vi "addmmWaveRefnums.vi"(8 "error in (no error)":errorcluster, 9 "mmWave motion ctrls":T1, 11 "UI ExecutionCtrls in":refnum<class "UI ExecutionCtrls.lvclass">) -> (0 "error out":errorcluster, 3 "UI ExecutionCtrls out":refnum<class "UI ExecutionCtrls.lvclass">)   [LabVIEW 2018, in "UI ExecutionCtrls.lvclass"]
uses:
  UI ExecutionCtrls.lvclass
  mmWaveMotionCrtlRefs.ctl
  UI ExecutionCtrls.lvclass/UI ExecutionCtrls.ctl
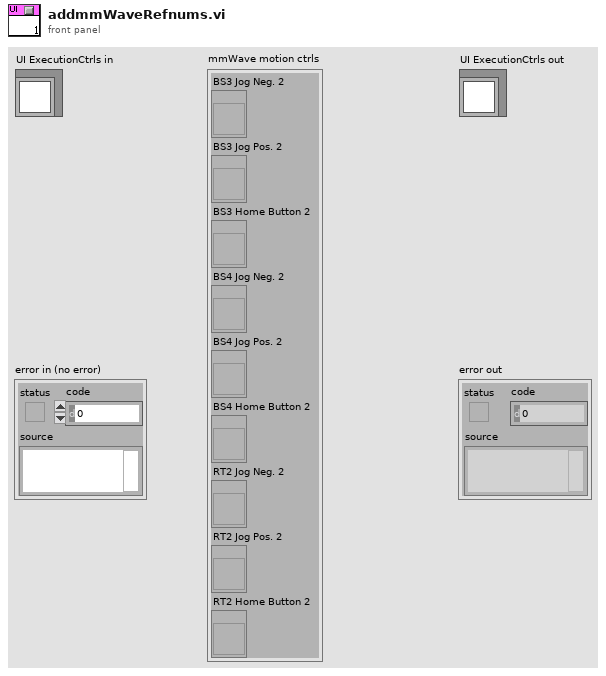
[diagram p1: front panel]
types:
  T1 = typedef "mmWaveMotionCrtlRefs.ctl" = cluster{"BS3 Jog Neg. 2":refnum<vi>, "BS3 Jog Pos. 2":refnum<vi>, "BS3 Home Button 2":refnum<vi>, "BS4 Jog Neg. 2":refnum<vi>, "BS4 Jog Pos. 2":refnum<vi>, "BS4 Home Button 2":refnum<vi>, "RT2 Jog Neg. 2":refnum<vi>, "RT2 Jog Pos. 2":refnum<vi>, "RT2 Home Button 2":refnum<vi>}
  T2 = enum8{"Enabled", "Disabled", "Disabled and Grayed Out"}
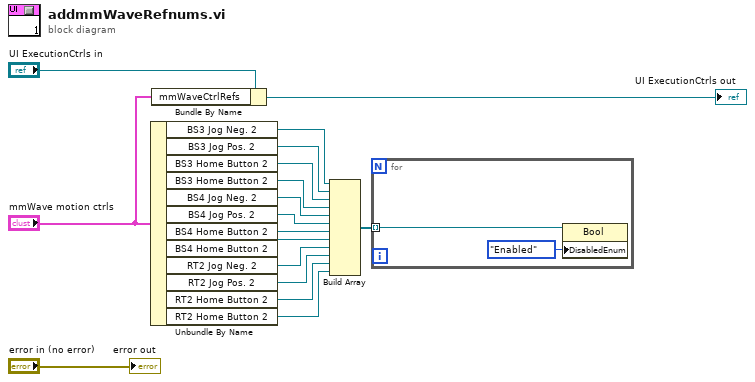
[diagram p0: block diagram]
diagram:
  n1 = Unbundle By Name("mmWave motion ctrls") -> ("BS3 Jog Neg. 2"=w13:refnum<vi>, "BS3 Jog Pos. 2"=w12:refnum<vi>, "BS3 Home Button 2"=w11:refnum<vi>, "BS3 Home Button 2"=w1:refnum<vi>, "BS4 Jog Neg. 2"=w10:refnum<vi>, "BS4 Jog Pos. 2"=w9:refnum<vi>, "BS4 Home Button 2"=w8:refnum<vi>, "BS4 Home Button 2"=w2:refnum<vi>, "RT2 Jog Neg. 2"=w7:refnum<vi>, "RT2 Jog Pos. 2"=w6:refnum<vi>, "RT2 Home Button 2"=w5:refnum<vi>, "RT2 Home Button 2"=w4:refnum<vi>)
  n2 = Bundle By Name(cluster="UI ExecutionCtrls in", "mmWaveCtrlRefs"="mmWave motion ctrls") -> (→"UI ExecutionCtrls out":refnum<class "UI ExecutionCtrls.lvclass">)
  n3 = Build Array(w13, w12, w11, w1, w10, w9, w8, w2, w7, w6, w5, w4) -> (w3:refnum<vi>[])
  n4 = for {
    tunnel: w3 -> [w19] mode=indexing
    n5 = property class="Bool"(reference=w19, "DisabledEnum"=T2."Enabled" ("Disabled")) -> ()  [unwired: 1 in, 2 out]
  }
  "error out" <- "error in (no error)"
